vi "UI_Show_Hide_Strings.vi"(8 "error in (no error)":errorcluster, 10 "Show ?":bool, 11 "Strings":refnum<vi>[](array[refnum])) -> (0 "error out":errorcluster caption="sortie d'erreur")   [LabVIEW 2018]
doc: "Définit toutes les commandes du tableau en entrée à la valeur \"État Activé\"."
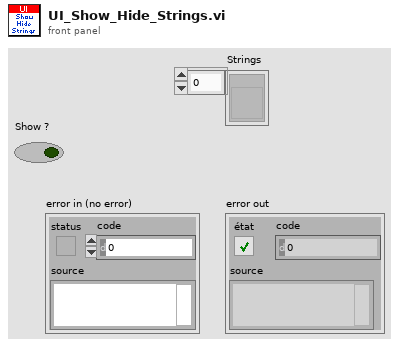
[diagram p1: front panel]
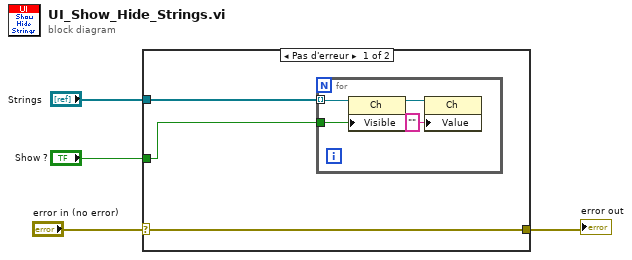
[diagram p0: block diagram]
diagram:
  n1 = case shown="Pas d'erreur" "error in (no error)" {
    selector: "error in (no error)" -> [w7 w12]
    tunnel: "Show ?" -> [w5 _]
    tunnel: [w7 w12] -> w2
    tunnel: "Strings" -> [w6 _]
    frame No Error {
      n2 = for {
        tunnel: w6 -> [w11] mode=indexing
        tunnel: w5 -> [w10]
        n3 = property class="Ch"(reference=w11, "Visible"=w10) -> (reference out=w9:refnum<vi>)  [unwired: 1 in, 1 out]
        n4 = property class="Ch"(reference=w9, "Value"="" ("Valeur")) -> ()  [unwired: 1 in, 2 out]
      }
    }
    frame Error {
    }
  }
  "error out" <- w2
